vi "ParamArray.vi"(9 "Step Size":dbl, 10 "Final Value":dbl, 11 "Initial Value":dbl) -> (3 "Array":dbl[](array[numeric]))   [LabVIEW 2013]
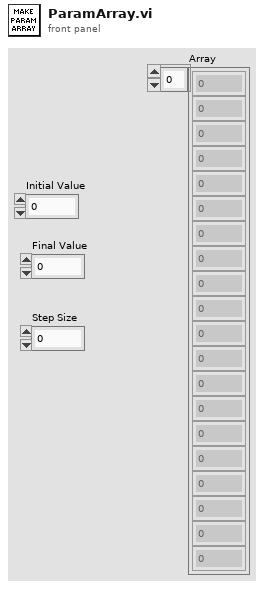
[diagram p1: front panel]
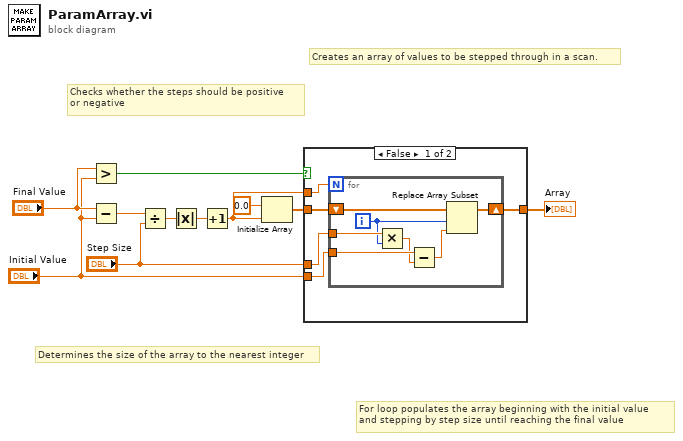
[diagram p0: block diagram]
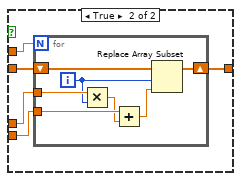
[diagram p2: hidden frame]
diagram:
  # "For loop populates the array beginning with the initial value\nand stepping by step size until reaching the final value"
  # "Determines the size of the array to the nearest integer"
  # "Checks whether the steps should be positive\nor negative"
  # "Creates an array of values to be stepped through in a scan."
  n1 = Greater?(x="Final Value", y="Initial Value") -> (0:w7:bool)
  n2 = Subtract(x="Final Value", y="Initial Value") -> (x-y=w11:dbl)
  n3 = Divide(x=w11, y="Step Size") -> (x/y=w9:dbl)
  n4 = Absolute Value(x=w9) -> (abs(x)=w2:dbl)
  n5 = Increment(x=w2) -> (x+1=w1:dbl)
  n6 = Initialize Array(0.0 ("element"), w1) -> (w6:dbl[])
  n7 = case shown="False" w7 {
    tunnel: w6 -> [w14 w28]
    tunnel: w1 -> [w16 w27]
    tunnel: "Step Size" -> [w13 w26]
    tunnel: "Initial Value" -> [w12 w25]
    tunnel: [w15 w24] -> w3
    frame False {
      n8 = for {
        N: w16 -> [_]
        shift-right: [w17] -> w15
        shift-left: w14 -> [w18]
        tunnel: w13 -> [w23]
        tunnel: w12 -> [w22]
        i -> [w20]
        n9 = Multiply(x=w23, y=w20) -> (x*y=w21:dbl)
        n10 = Subtract(x=w22, y=w21) -> (x-y=w19:dbl)
        n11 = Replace Array Subset(array=w18, new element=w19, index=w20) -> (w17:dbl[])
      }
    }
    frame True {
      n12 = for {
        N: w27 -> [_]
        shift-right: [w34] -> w24
        shift-left: w28 -> [w35]
        tunnel: w26 -> [w33]
        tunnel: w25 -> [w32]
        i -> [w29]
        n13 = Multiply(x=w33, y=w29) -> (x*y=w31:dbl)
        n14 = Add(x=w32, y=w31) -> (x+y=w30:dbl)
        n15 = Replace Array Subset(array=w35, new element=w30, index=w29) -> (w34:dbl[])
      }
    }
  }
  "Array" <- w3
